vi "Test TimeOUT.vi"(0 "OLD Time":u32, 3 "TimeOut ms":u32) -> (14 "Timeout ?":bool, 15 "NEW Time":u32, 17 "Temps restant":u32, 18 "Chaîne":string, 19 "valeur de l'horloge en ms":u32)   [LabVIEW 2020, in "Library Commun.lvlib"]
uses:
  Library Commun.lvlib
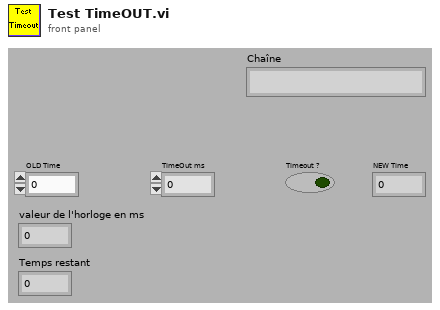
[diagram p1: front panel]
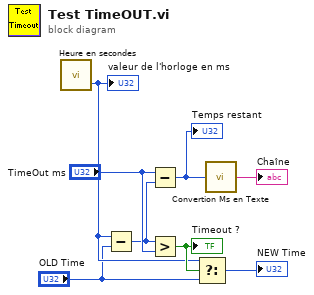
[diagram p0: block diagram]
diagram:
  n1 = call "Heure en secondes.vi"() -> ("Heure en milisecondes"=w3:u32)  [unwired: 2 in, 1 out]
  "valeur de l'horloge en ms" <- w3
  n2 = Subtract(x=w3, y="OLD Time") -> (x-y=w5:u32)
  n3 = Subtract(x="TimeOut ms", y=w5) -> (x-y=w7:u32)
  "Temps restant" <- w7
  n4 = Greater?(x=w5, y="TimeOut ms") -> (0:w4:bool)
  "Timeout ?" <- w4
  n5 = Select(t=w3, s=w4, f="OLD Time") -> (s? t:f=→"NEW Time":u32)
  n6 = call "Convertion Ms en Texte.vi"("Numérique"=w7) -> ("Chaîne"=→"Chaîne":string)
